vi "Run Client.vi"(8 "error in":errorcluster, 10 "pin map context":T1, 11 "measurement configuration":T3) -> (0 "error out":errorcluster, 3 "measurement results":T2)   [LabVIEW 2021, in "Measurement Client Template.lvlib"]
doc: "<B>Run Client.vi</B> is a wrapper to demonstrate the working of Measurement Plug-In Client. It performs the following functions:\n- Create a client for the measurement service\n- Run the measurement logic and display the results\n- Close the client connection."
uses:
  Measurement Client Template.lvlib
  controls/Measurement Configuration.ctl
  controls/Measurement Results.ctl
  <vilib>/gRPC/Generated APIs/ni/measurementlink/measurement/v2/Measurement Service Client V2/RPC Messages/ni_measurementlink_PinMapContext.ctl
  <vilib>/gRPC/Generated APIs/ni/measurementlink/measurement/v2/Measurement Service Client V2/Measurement Service Client V2.lvlib
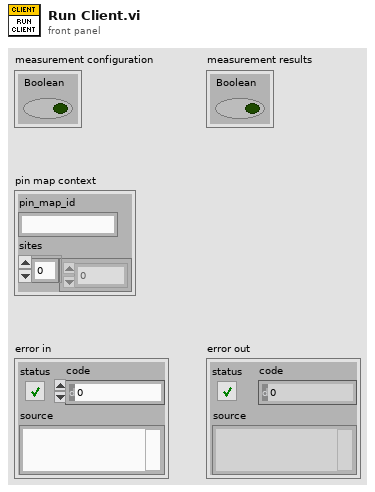
[diagram p1: front panel]
types:
  T1 = typedef "Measurement Service Client V2.lvlib/ni_measurementlink_PinMapContext.ctl" = cluster{"pin_map_id":string, "sites":i32[]}
  T2 = typedef "Measurement Client Template.lvlib/Measurement Results.ctl" = cluster{"Boolean":bool}
  T3 = typedef "Measurement Client Template.lvlib/Measurement Configuration.ctl" = cluster{"Boolean":bool}
  T4 = typedef "grpc-lvsupport-release.lvlib/grpcId.ctl" = u64
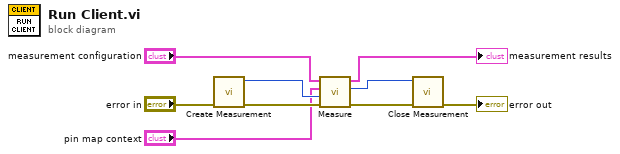
[diagram p0: block diagram]
diagram:
  n1 = call "Create Measurement.vi"("error in"="error in") -> ("error out"=w9:errorcluster, "gRPCid out"=w5:T4)  [unwired: 9 in]
  n2 = call "Measure.vi"("error in"=w9, "gRPCid in"=w5, "pin map context"="pin map context", "measurement configuration"="measurement configuration") -> ("error out"=w8:errorcluster, "gRPCid out"=w2:u64, "measurement results"=→"measurement results":T2)  [unwired: 5 in]
  n3 = call "Close Measurement.vi"("error in"=w8, "gRPCid in"=w2) -> ("error out"=→"error out":errorcluster)  [unwired: 9 in]
